vi "setFontToDocument.vi"(8 "error in (no error)":errorcluster, 11 "xwpfRun in":refnum<class "xwpfRun.lvclass">) -> (0 "error out":errorcluster, 3 "xwpfRun out":refnum<class "xwpfRun.lvclass">)   [LabVIEW 2017, in "Word_Specific.lvlib" / "xwpfRun.lvclass"]
uses:
  xwpfRun.lvclass
  xwpfRun.lvclass/xwpfRun.ctl
  C:/Users/Neo/Desktop/Dev_Tools_BR/LabVIEW_NPOI/lib/NPOI 2.1.1/NPOI.OOXML.dll
  lib/NPOI 2.1.1/NPOI.OOXML.dll
  Styles/Style/Style.lvclass
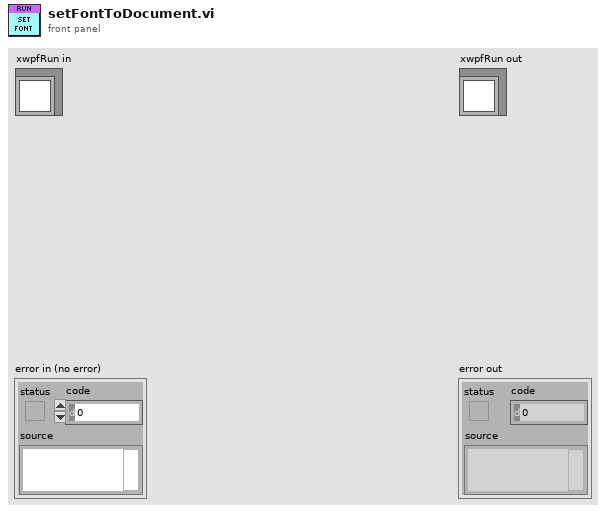
[diagram p1: front panel]
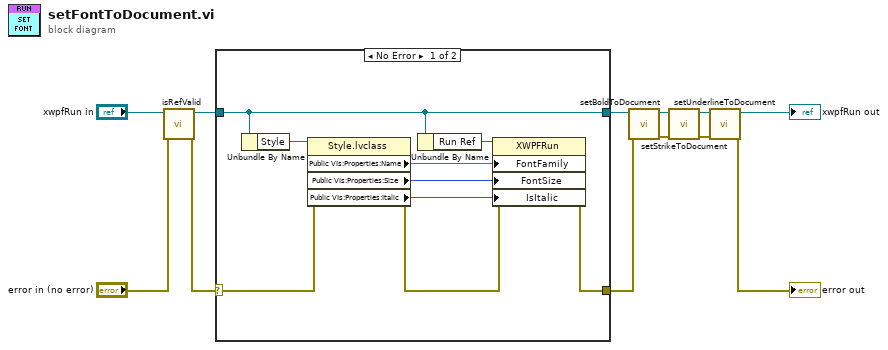
[diagram p0: block diagram]
diagram:
  n1 = call-dynamic "isRefValid.vi"("error in (no error)"="error in (no error)", "xwpfRun in"="xwpfRun in") -> ("error out"=w9:errorcluster, "xwpfRun out"=w11:refnum<class "xwpfRun.lvclass">)  [unwired: 8 in]
  n2 = case shown="No Error" w9 {
    selector: w9 -> [w19 w23]
    tunnel: [w17 w23] -> w2
    tunnel: [w16 w22] -> w8
    tunnel: w11 -> [w16 w22]
    frame No Error {
      n3 = Unbundle By Name(w16) -> ("Style"=w20:refnum<class "Style.lvclass">)
      n4 = property class="Style.lvclass"(reference=w20, error in=w19) -> (error out=w18:errorcluster, "Public VIs:Properties:Name"=w15:string, "Public VIs:Properties:Size"=w14:i32, "Public VIs:Properties:Italic"=w13:bool)  [unwired: 1 out]
      n5 = Unbundle By Name(w16) -> ("Run Ref"=w21:refnum<k24>)
      n6 = property class="XWPFRun"(reference=w21, error in=w18, "FontFamily"=w15, "FontSize"=w14, "IsItalic"=w13) -> (error out=w17:errorcluster)  [unwired: 1 out]
    }
    frame Error {
    }
  }
  n7 = call "setBoldToDocument.vi"("error in (no error)"=w2, "xwpfRun in"=w8) -> ("error out"=w3:errorcluster, "xwpfRun out"=w7:refnum<class "xwpfRun.lvclass">)  [unwired: 8 in]
  n8 = call "setStrikeToDocument.vi"("error in (no error)"=w3, "xwpfRun in"=w7) -> ("error out"=w4:errorcluster, "xwpfRun out"=w6:refnum<class "xwpfRun.lvclass">)  [unwired: 8 in]
  n9 = call "setUnderlineToDocument.vi"("error in (no error)"=w4, "xwpfRun in"=w6) -> ("error out"=→"error out":errorcluster, "xwpfRun out"=→"xwpfRun out":refnum<class "xwpfRun.lvclass">)  [unwired: 8 in]
